vi "cerebellum.vi"   [LabVIEW 2013]
uses:
  Cerebellum/Cerebellum.lvclass
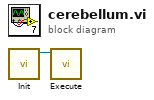
[diagram p0: block diagram]
diagram:
  n1 = call "Init.vi"() -> ("Scene Object Out"=w1:refnum<vi>)  [unwired: 9 in, 2 out]
  n2 = call "Execute.vi"("Cerebellum in"=w1) -> ()  [unwired: 10 in, 1 out]
